vi "Export.vi"(8 "error in (no error)":errorcluster, 10 "IExporter":refnum<class "IExporter.lvclass">, 11 "CRuleList in":refnum<class "CRuleList.lvclass">) -> (0 "error out":errorcluster, 3 "CRuleList out":refnum<class "CRuleList.lvclass">)   [LabVIEW 2020, in "DependencyInspection.lvlib" / "CRuleList.lvclass"]
uses:
  CRuleList.lvclass
  obj/Addons/ExtensionInterfaces.lvlibp/IExporter/IExporter.lvclass
  obj/Addons/ExtensionInterfaces.lvlibp/IExporter/ExportType.ctl
  obj/Addons/LabVIEWObjectInterfaces.lvlibp/LabVIEWObjectInterfaces/IDependencyItemRule/IDependencyItemRule.lvclass
  E:/Repos/LVDependencyInspector/obj/Addons/LabVIEWObjectInterfaces.lvlibp/LabVIEWObjectInterfaces/ILabVIEWItem/ILabVIEWItem.lvclass
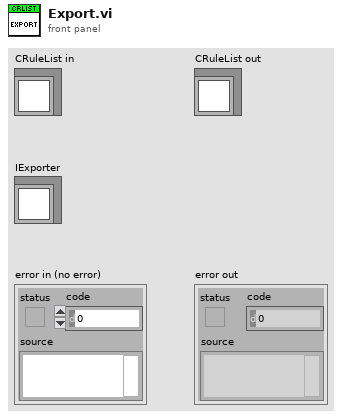
[diagram p1: front panel]
types:
  T1 = typedef "ExtensionInterfaces.lvlibp/IExporter.lvclass/ExportType.ctl" = enum16{"Dependencies", "Rules", "Invalid dependencies", "Concessions", "Undeclared"}
  T2 = typedef "DependencyInspection.lvlib/CRuleList.lvclass/RuleList.ctl" = map{string, refnum<class "IDependencyItemRule.lvclass">}
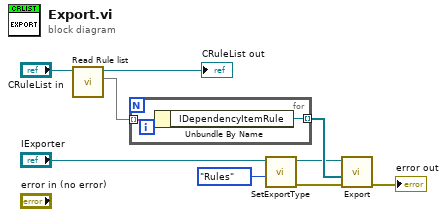
[diagram p0: block diagram]
diagram:
  n1 = call-dynamic "Read Rule list.vi"("CRuleList in"="CRuleList in") -> ("Rule List"=w7:T2, "CRuleList out"=→"CRuleList out":refnum<class "CRuleList.lvclass">)  [unwired: 9 in]
  n2 = for {
    tunnel: w7 -> [w11] mode=indexing
    tunnel: [w10] -> w6 mode=indexing
    n3 = Unbundle By Name(w11) -> ("IDependencyItemRule"=w10:refnum<class "IDependencyItemRule.lvclass">)
  }
  n4 = call-dynamic "SetExportType.vi"("Export type"=ExportType."Rules", "IExporter in"="IExporter") -> ("error out"=w1:errorcluster, "IExporter out"=w2:refnum<class "IExporter.lvclass">)  [unwired: 8 in]
  n5 = call-dynamic "Export.vi"("error in (no error)"=w1, "Items"=w6, "IExporter in"=w2) -> ("error out"=→"error out":errorcluster)  [unwired: 7 in, 1 out]
